vi "StreamDAQ.vi"(5 "control data type":variant, 7 "Logging Queue":refnum<queue>, 9 "StreamTypeDef":T1, 11 "error in":errorcluster) -> (4 "control data out":variant, 10 "StreamTypeDef":T1, 15 "error out":errorcluster)   [LabVIEW 2024]
uses:
  Control/StreamTypeDef.ctl
  Control/streamIO_states.ctl
panel:
  in  "Stream Data Type":dbl[][](array[numeric])
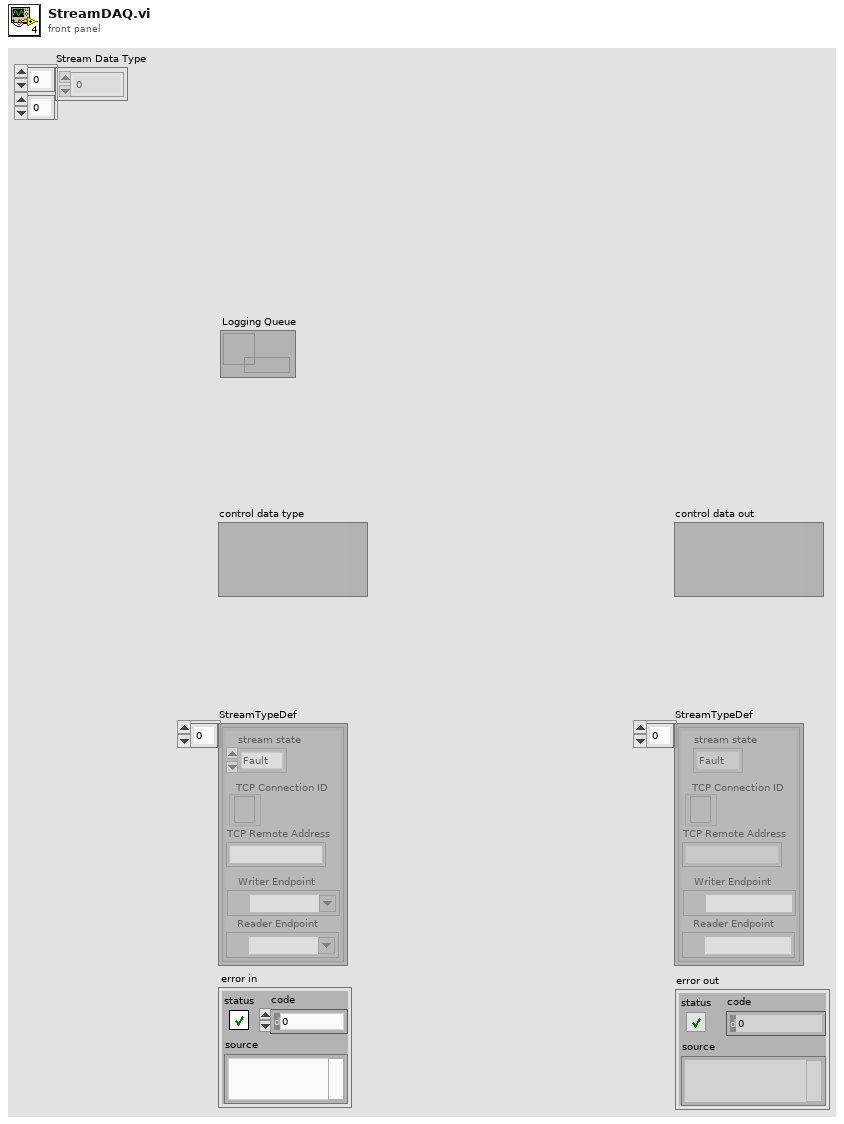
[diagram p1: front panel]
types:
  T1 = typedef "StreamTypeDef.ctl" = cluster{"stream state":T2, "TCP Remote Address":string, "TCP Connection ID":refnum<k5>, "Reader Endpoint":refnum<k21>, "Writer Endpoint":refnum<k21>}[]
  T2 = typedef "streamIO_states.ctl" = enum16{"Fault", "Initilize", "Stream", "Close"}
  T3 = cluster{"stream state":T2, "TCP Remote Address":string, "TCP Connection ID":refnum<k5>, "Reader Endpoint":refnum<k21>, "Writer Endpoint":refnum<k21>}
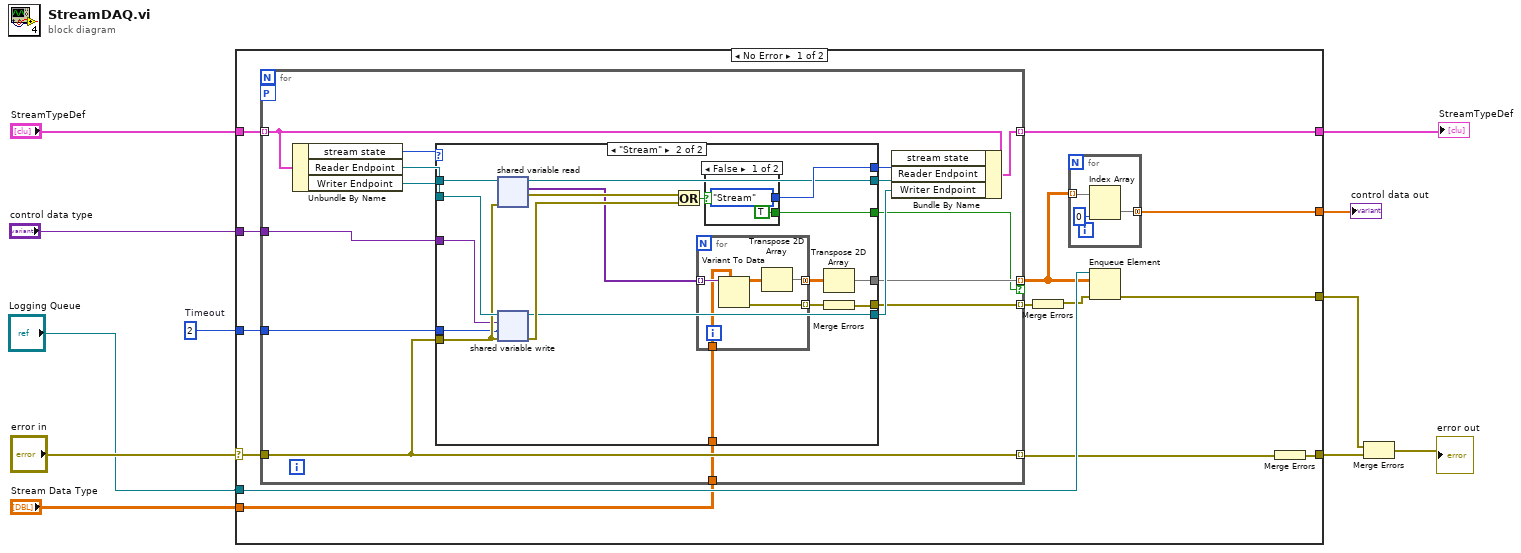
[diagram p0: block diagram]
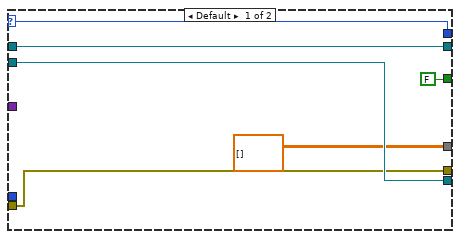
[diagram p2: hidden frame]
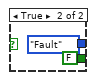
[diagram p3: hidden frame]
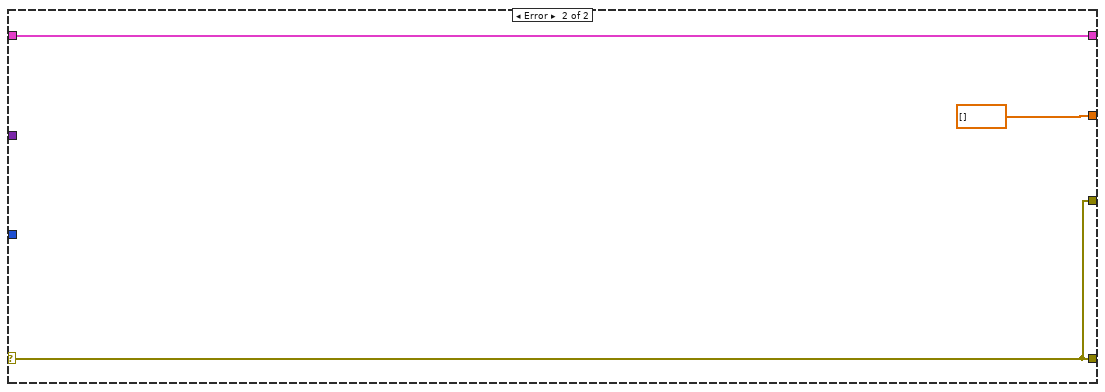
[diagram p4: hidden frame]
diagram:
  w6 = 2  # Timeout
  n1 = case shown="No Error" "error in" {
    selector: "error in" -> [w21 w79]
    tunnel: "StreamTypeDef" -> [w25 w78]
    tunnel: [w24 w78] -> w10
    tunnel: [w15 w79] -> w9
    tunnel: "control data type" -> [w23 _]
    tunnel: w6 -> [w22 _]
    tunnel: "Logging Queue" -> [w20 _]
    tunnel: "Stream Data Type" -> [w19 _]
    tunnel: [w16 w79] -> w2
    tunnel: [w12 dbl[] []] -> w1
    frame No Error {
      n2 = for {
        workers-P: _ -> [_]
        tunnel: w25 -> [w38] mode=indexing
        tunnel: [w37] -> w24 mode=indexing
        tunnel: [w40] -> w14 mode=indexing
        tunnel: w21 -> [w40]
        tunnel: w23 -> [w39]
        tunnel: w22 -> [w33]
        tunnel: w19 -> [w32]
        tunnel: [w31] -> w13 mode=indexing if=w29
        tunnel: [w30] -> w17 mode=indexing
        n3 = Unbundle By Name(w38) -> ("stream state"=w43:T2, "Reader Endpoint"=w42:refnum<k21>, "Writer Endpoint"=w41:refnum<k21>)
        n4 = case shown="\"Stream\"" w43 {
          selector: w43 -> [w47 _]
          tunnel: w42 -> [w49 w67]
          tunnel: w41 -> [w48 w66]
          tunnel: w40 -> [w45 w65]
          tunnel: w39 -> [_ w64]
          tunnel: [w47 w60] -> w36
          tunnel: [w49 w59] -> w35
          tunnel: [w48 w58] -> w34
          tunnel: w33 -> [_ w57]
          tunnel: w32 -> [_ w55]
          tunnel: [dbl[][] [] w53] -> w31
          tunnel: [w45 w52] -> w30
          tunnel: [FALSE w50] -> w29
          frame Default {
          }
          frame "Stream" {
            n5 = shared-variable-read(w67, w65) -> (w59:refnum<k21>, w62:errorcluster, w56:variant[])  [unwired: 2 in, 1 out]
            n6 = shared-variable-write(w66, w65, w64, w57) -> (w58:refnum<k21>, w61:errorcluster)  [unwired: 1 out]
            n7 = Or(x=w62, y=w61) -> (x .or. y?=w63:bool)
            n8 = for {
              tunnel: w56 -> [w72] mode=indexing
              tunnel: w55 -> [w71]
              tunnel: [w69] -> w54 mode=concatenating
              tunnel: [w68] -> w51 mode=indexing
              n9 = Variant To Data(type=w71, Variant=w72) -> (data=w70:dbl[][], error out=w68:errorcluster)  [unwired: 1 in]
              n10 = Transpose 2D Array(2D array=w70) -> (transposed array=w69:dbl[][])
            }
            n11 = case shown="False" w63 {
              tunnel: [streamIO_states."Stream" ("stream state") streamIO_states."Fault" ("stream state")] -> w60
              tunnel: [TRUE FALSE] -> w50
              frame False {
              }
              frame True {
              }
            }
            n12 = Transpose 2D Array(2D array=w54) -> (transposed array=w53:dbl[][])
            n13 = Merge Errors(w51) -> (w52:errorcluster)
          }
        }
        n14 = Bundle By Name(cluster=w38, "stream state"=w36, "Reader Endpoint"=w35, "Writer Endpoint"=w34) -> (w37:T3)
      }
      n15 = Merge Errors(w17) -> (w18:errorcluster)
      n16 = for {
        tunnel: w13 -> [w28] mode=indexing
        tunnel: [w26] -> w12 mode=concatenating
        n17 = Index Array(array=w28, index (col)=0) -> (element=w26:dbl[])  [unwired: 1 in]
      }
      n18 = Enqueue Element(queue=w20, element=w13, error in (no error)=w18) -> (error out=w16:errorcluster)  [unwired: 1 in, 2 out]
      n19 = Merge Errors(w14) -> (w15:errorcluster)
    }
    frame Error {
    }
  }
  "StreamTypeDef" <- w10
  "control data out" <- w1
  n20 = Merge Errors(w2, w9) -> (→"error out":errorcluster)
